vi "pattern_match+matching_decay+direction&boudning_box.vi"(0 "Imaginea":path, 1 "Template":path) -> (13 "y 2":sgl, 14 "Directia":i32, 15 "x":sgl, 17 "y":sgl, 18 "x 2":sgl, 19 "Image":T1(plugin-control))   [LabVIEW 2015]
panel:
  out "Angle":sgl
  out "element":T2
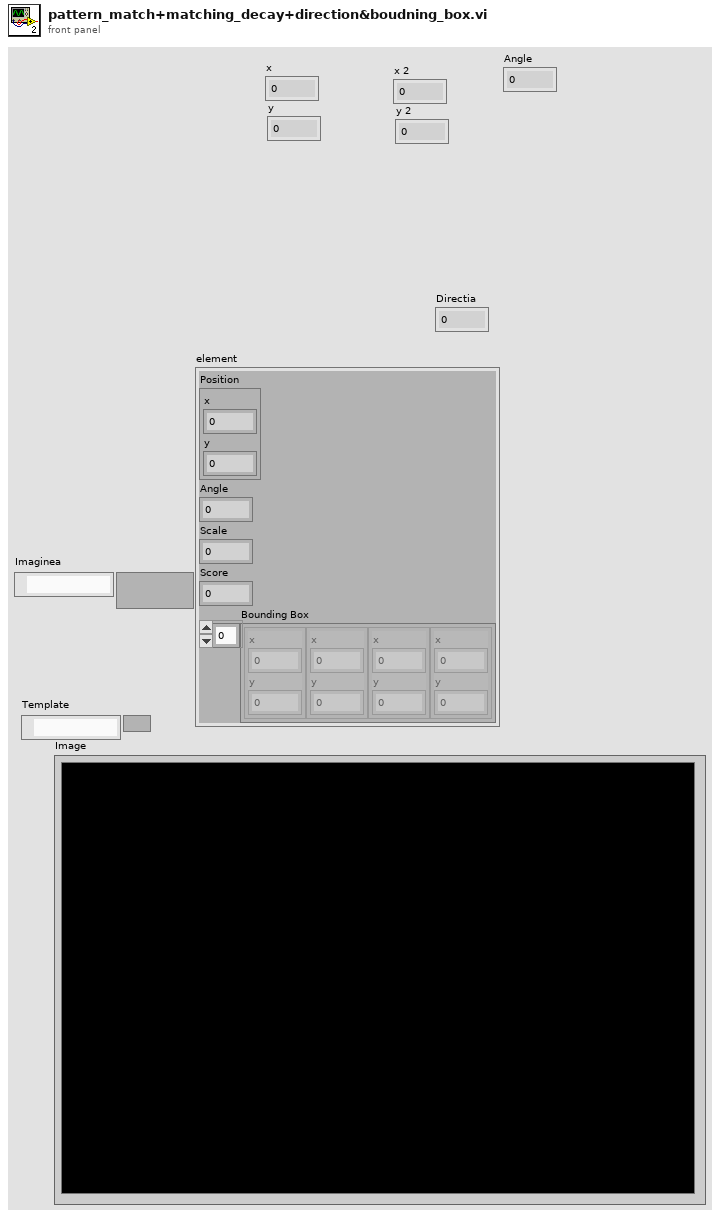
[diagram p1: front panel]
types:
  T1 = typedef "IMAQ Image.ctl" = refnum<image>
  T2 = cluster{"Position":cluster{"x":sgl, "y":sgl}, "Angle":sgl, "Scale":sgl, "Score":sgl, "Bounding Box":cluster{"x":sgl, "y":sgl}[]}
  T3 = cluster{"Position":cluster{"x":sgl, "y":sgl}, "Angle":sgl, "Scale":sgl, "Score":sgl, "Bounding Box":cluster{"x":sgl, "y":sgl}[]}[]
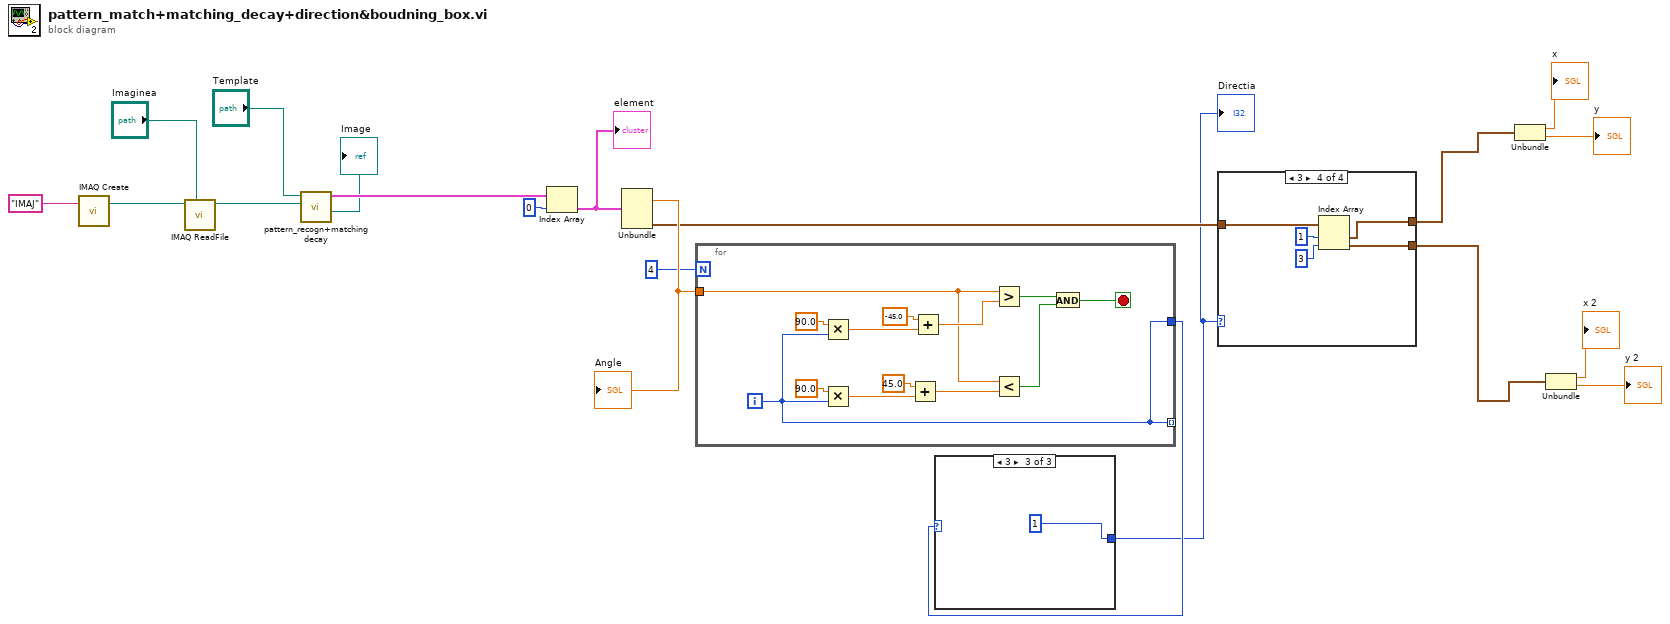
[diagram p0: block diagram]
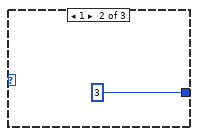
[diagram p3: hidden frame]
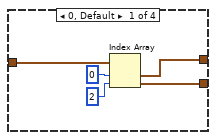
[diagram p4: hidden frame]
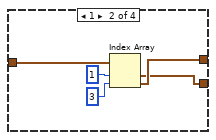
[diagram p5: hidden frame]
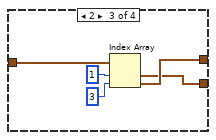
[diagram p6: hidden frame]
diagram:
  n1 = call "IMAQ Create"("Image Name"="IMAJ") -> ("New Image"=w20:T1)  [unwired: 4 in, 1 out]
  n2 = call "IMAQ ReadFile"("File Path"="Imaginea", "Image"=w20) -> ("Image Out"=w17:T1)  [unwired: 5 in, 4 out]
  n3 = call "pattern_recogn+matching decay.vi"("Image Out"=w17, "Path 3"="Template") -> ("Image"=→"Image":T1, "Matches (pixel)"=w15:T3)  [unwired: 7 in, 1 out]
  n4 = Index Array(array=w15, index=0) -> (element=w11:T2)
  "element" <- w11
  n5 = Unbundle(w11) -> ("Angle"=w13:sgl, "Bounding Box"=w10:cluster{"x":sgl, "y":sgl}[])  [unwired: 3 out]
  "Angle" <- w13
  n6 = for {
    N: 4 -> [_]
    tunnel: w13 -> [w27]
    tunnel: [w22] -> w3
    tunnel: [w22] -> _ mode=indexing
    i -> [w22]
    stop <- w24 stop-if-true
    n7 = Multiply(x=sgl 90.0, y=w22) -> (x*y=w31:sgl)
    n8 = Multiply(x=sgl 90.0, y=w22) -> (x*y=w21:sgl)
    n9 = Add(x=sgl 45.0, y=w21) -> (x+y=w28:sgl)
    n10 = Add(x=sgl -45.0, y=w31) -> (x+y=w30:sgl)
    n11 = Greater?(x=w27, y=w30) -> (0:w26:bool)
    n12 = Less?(x=w27, y=w28) -> (x < y?=w25:bool)
    n13 = And(x=w26, y=w25) -> (x .and. y?=w24:bool)
  }
  n14 = case shown="3" w3 {
    selector: w3 -> [w34 _ _]
    tunnel: [w34 3 1] -> w2
    frame 0, Default {
    }
    frame 1 {
    }
    frame 3 {
    }
  }
  "Directia" <- w2
  n15 = case shown="3" w2 {
    tunnel: w10 -> [w41 w44 w49 w54]
    tunnel: [w38 w43 w48 w53] -> w9
    tunnel: [w37 w42 w47 w52] -> w4
    frame 0, Default {
      n16 = Index Array(array=w41, index #1=0 ("index"), index #2=2 ("index")) -> (element #1=w38:cluster{"x":sgl, "y":sgl}, element #2=w37:cluster{"x":sgl, "y":sgl})
    }
    frame 1 {
      n17 = Index Array(array=w44, index #1=1 ("index"), index #2=3 ("index")) -> (element #1=w42:cluster{"x":sgl, "y":sgl}, element #2=w43:cluster{"x":sgl, "y":sgl})
    }
    frame 2 {
      n18 = Index Array(array=w49, index #1=1 ("index"), index #2=3 ("index")) -> (element #1=w47:cluster{"x":sgl, "y":sgl}, element #2=w48:cluster{"x":sgl, "y":sgl})
    }
    frame 3 {
      n19 = Index Array(array=w54, index #1=1 ("index"), index #2=3 ("index")) -> (element #1=w53:cluster{"x":sgl, "y":sgl}, element #2=w52:cluster{"x":sgl, "y":sgl})
    }
  }
  n20 = Unbundle(w9) -> ("x"=→"x":sgl, "y"=→"y":sgl)
  n21 = Unbundle(w4) -> ("x"=→"x 2":sgl, "y"=→"y 2":sgl)
